vi "DetectorReadData.vi"   [LabVIEW 2012, in "Microscope.lvclass"]
uses:
  classes/Microscope.lvclass
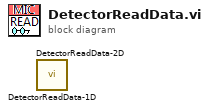
[diagram p0: block diagram]
diagram:
  n1 = call "DetectorReadData-1D.vi"() -> ()  [unwired: 17 in, 3 out]
  n2 = call "DetectorReadData-2D.vi"() -> ()  [unwired: 17 in, 3 out]
